vi "AlliGator Register Control Events.vi"(8 "Error In":errorcluster, 11 "AlliGator Control References":T2) -> (0 "Error Out":errorcluster, 3 "AlliGator Events Registration":T1)   [LabVIEW 2021, in "AlliGator GUI.lvlib"]
doc: "Registers user events for controls on the main AlliGator window."
uses:
  AlliGator GUI.lvlib
  AlliGator Registered Events Ctrl Refnums.ctl
  AlliGator Events Registration.ctl
  Settings/AlliGator Settings Event.ctl
  Settings/AlliGator Settings Window Messages.ctl
  Phasor Plot Color Map/AlliGator Phasor Color Map User Event List.ctl
  Graphs/XY Graph/XY Graph Refnum.ctl
  Settings/AlliGator Settings.lvlib
  Phasor Plot Color Map/AlliGator Phasor Plot Color Map.lvlib
  Phasor Plot/AlliGator Phasor Plot.lvlib
  Graphs/XY Graph/XY Graph Add-Ons.lvlib
panel:
  # "see the AlliGator License on the block diagram (Ctrl+E or Window:Show Block Diagram)"
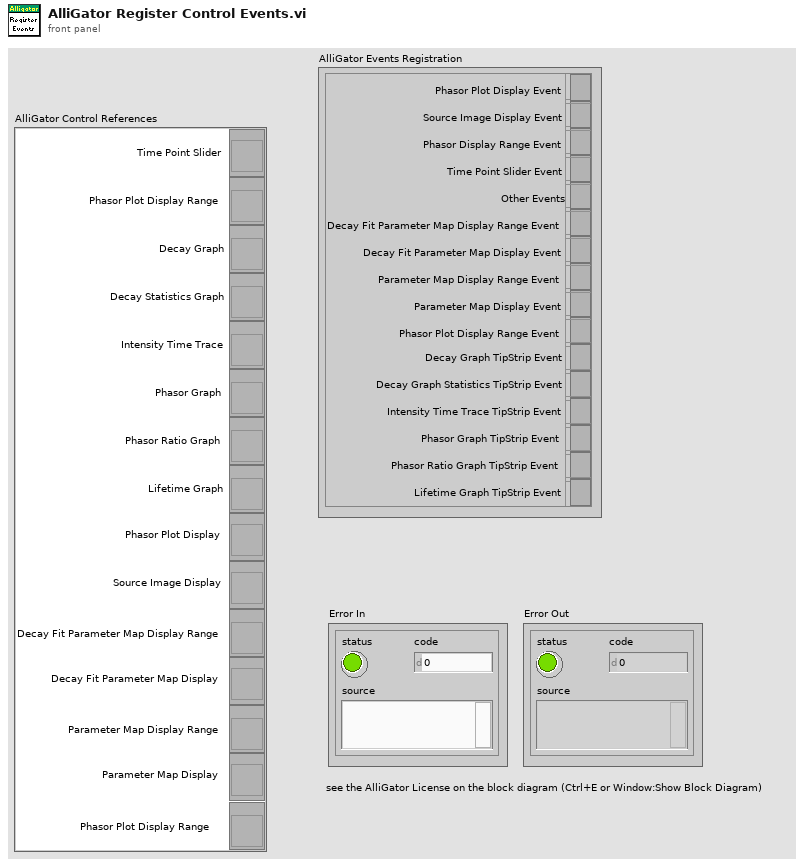
[diagram p1: front panel]
types:
  T1 = typedef "AlliGator GUI.lvlib/AlliGator Events Registration.ctl" = cluster{"Phasor Plot Display Event":refnum<event-registration>, "Source Image Display Event":refnum<event-registration>, "Phasor Display Range Event":refnum<event-registration>, "Time Point Slider Event":refnum<event-registration>, "Other Events":refnum<event-registration>, "Decay Fit Parameter Map Display Range Event":refnum<event-registration>, "Decay Fit Parameter Map Display Event":refnum<event-registration>, "Parameter Map Display Range Event":refnum<event-registration>, "Parameter Map Display Event":refnum<event-registration>, "Phasor Plot Display Range Event":refnum<event-registration>, "Decay Graph TipStrip Event":refnum<event-registration>, "Decay Graph Statistics TipStrip Event":refnum<event-registration>, "Intensity Time Trace TipStrip Event":refnum<event-registration>, "Phasor Graph TipStrip Event":refnum<event-registration>, "Phasor Ratio Graph TipStrip Event":refnum<event-registration>, "Lifetime Graph TipStrip Event":refnum<event-registration>}
  T2 = typedef "AlliGator GUI.lvlib/AlliGator Registered Events Ctrl Refnums.ctl" = cluster{"Time Point Slider":refnum<vi>, "Phasor Plot Display Range":refnum<vi>, "Decay Graph":refnum<vi>, "Decay Statistics Graph":refnum<vi>, "Intensity Time Trace":refnum<vi>, "Phasor Graph":refnum<vi>, "Phasor Ratio Graph":refnum<vi>, "Lifetime Graph":refnum<vi>, "Phasor Plot Display":refnum<vi>, "Source Image Display":refnum<vi>, "Decay Fit Parameter Map Display Range":refnum<vi>, "Decay Fit Parameter Map Display":refnum<vi>, "Parameter Map Display Range":refnum<vi>, "Parameter Map Display":refnum<vi>, "Phasor Plot Display Range":refnum<vi>}
  T3 = cluster{"Event Registration Refnum":refnum<event-registration>, "Event Registration Refnum":refnum<event-registration>, "Event Registration Refnum":refnum<event-registration>, "Event Registration Refnum":refnum<event-registration>, "Event Registration Refnum":refnum<event-registration>, "Event Registration Refnum":refnum<event-registration>, "Event Registration Refnum":refnum<event-registration>, "Event Registration Refnum":refnum<event-registration>, "Event Registration Refnum":refnum<event-registration>, "Event Registration Refnum":refnum<event-registration>, "Event Registration Refnum":refnum<event-registration>, "Event Registration Refnum":refnum<event-registration>, "Event Registration Refnum":refnum<event-registration>, "Event Registration Refnum":refnum<event-registration>, "Event Registration Refnum":refnum<event-registration>, "Event Registration Refnum":refnum<event-registration>}
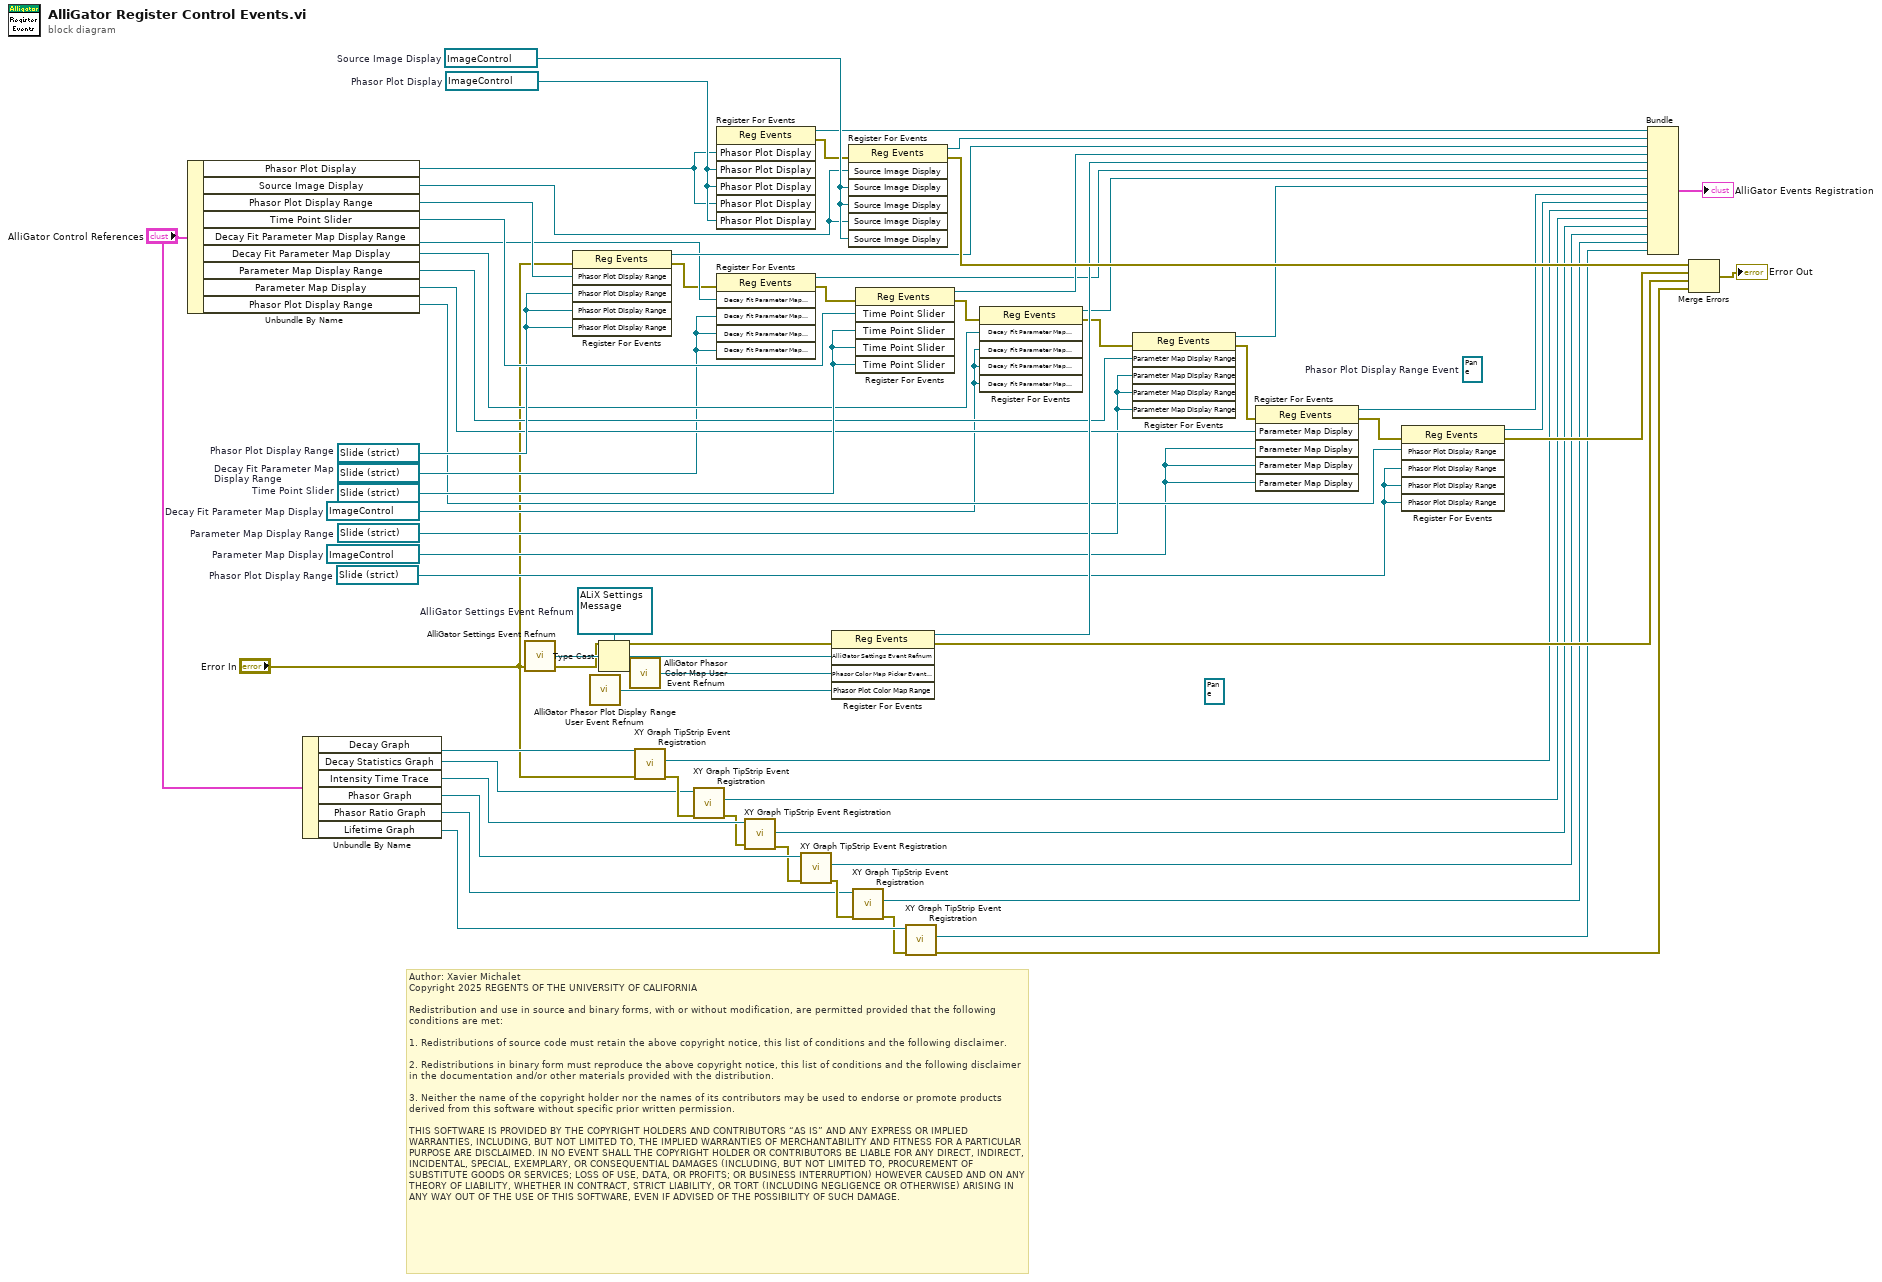
[diagram p0: block diagram]
diagram:
  (unwired) refnum<event-registration> refnum ("Decay Graph TipStrip Event")
  (unwired) refnum<event-registration> refnum  # Phasor Plot Display Range Event
  w25 = refnum<vi> refnum  # Phasor Plot Display Range
  w23 = refnum<vi> refnum  # Parameter Map Display
  w31 = refnum<vi> refnum  # Parameter Map Display Range
  w22 = refnum<vi> refnum  # Decay Fit Parameter Map Display
  w32 = refnum<vi> refnum  # Decay Fit Parameter Map Display Range
  w47 = refnum<vi> refnum  # Time Point Slider
  w48 = refnum<vi> refnum  # Phasor Plot Display Range
  w66 = refnum<user-event> refnum  # AlliGator Settings Event Refnum
  w62 = refnum<vi> refnum  # Source Image Display
  w63 = refnum<vi> refnum  # Phasor Plot Display
  # "Author: Xavier Michalet\nCopyright 2025 REGENTS OF THE UNIVERSITY OF CALIFORNIA\n\nRedistribution and use in source and binary forms, with or without modification, are permitted provided that the following conditions are met:\n\n1. Redistributions of source code must retain the above copyright notice, this list of conditions and the following disclaimer.\n\n2. Redistributions in binary form must reproduce the above copyright notice, this list of conditions and the following disclaimer in the documentation and/or other materials provided with the distribution.\n\n3. Neither the name of the copyright holder nor the names of its contributors may be used to endorse or promote products derived from this software without specific prior written permission.\n\nTHIS SOFTWARE IS PROVIDED BY THE COPYRIGHT HOLDERS AND CONTRIBUTORS “AS IS” AND ANY EXPRESS OR IMPLIED WARRANTIES, INCLUDING, BUT NOT LIMITED TO, THE IMPLIED WARRANTIES OF MERCHANTABILITY AND FITNESS FOR A PARTICULAR PURPOSE ARE DISCLAIMED. IN NO EVENT SHALL THE COPYRIGHT HOLDER OR CONTRIBUTORS BE LIABLE FOR ANY DIRECT, INDIRECT, INCIDENTAL, SPECIAL, EXEMPLARY, OR CONSEQUENTIAL DAMAGES (INCLUDING, BUT NOT LIMITED TO, PROCUREMENT OF SUBSTITUTE GOODS OR SERVICES; LOSS OF USE, DATA, OR PROFITS; OR BUSINESS INTERRUPTION) HOWEVER CAUSED AND ON ANY THEORY OF LIABILITY, WHETHER IN CONTRACT, STRICT LIABILITY, OR TORT (INCLUDING NEGLIGENCE OR OTHERWISE) ARISING IN ANY WAY OUT OF THE USE OF THIS SOFTWARE, EVEN IF ADVISED OF THE POSSIBILITY OF SUCH DAMAGE."
  n1 = Unbundle By Name("AlliGator Control References") -> ("Phasor Plot Display"=w40:refnum<vi>, "Source Image Display"=w41:refnum<vi>, "Phasor Plot Display Range"=w52:refnum<vi>, "Time Point Slider"=w50:refnum<vi>, "Decay Fit Parameter Map Display Range"=w45:refnum<vi>, "Decay Fit Parameter Map Display"=w38:refnum<vi>, "Parameter Map Display Range"=w34:refnum<vi>, "Parameter Map Display"=w35:refnum<vi>, "Phasor Plot Display Range"=w26:refnum<vi>)
  n2 = Unbundle By Name("AlliGator Control References") -> ("Decay Graph"=w20:refnum<vi>, "Decay Statistics Graph"=w15:refnum<vi>, "Intensity Time Trace"=w14:refnum<vi>, "Phasor Graph"=w13:refnum<vi>, "Phasor Ratio Graph"=w9:refnum<vi>, "Lifetime Graph"=w8:refnum<vi>)
  n3 = call "AlliGator Settings Event Refnum.vi"("Error In"="Error In") -> ("AlliGator Settings Event Refnum"=w65:refnum<user-event>, "Error Out"=w46:errorcluster)  [unwired: 7 in]
  n4 = register-events(error in="Error In", w52, w48, w48, w48) -> (reference out=w51:refnum<event-registration>, error out=w44:errorcluster)  [unwired: 1 in]
  n5 = call "AlliGator Phasor Plot Display Range User Event Refnum.vi"() -> ("Phasor Plot Color Map Range"=w57:refnum<user-event>)  [unwired: 9 in]
  n6 = Type Cast(type=w66, x=w65) -> (*(type *) &x=w59:refnum<user-event>)
  n7 = call "AlliGator Phasor Color Map User Event Refnum.vi"() -> ("Phasor Color Map Picker Event Refnum"=w58:refnum<user-event>)  [unwired: 9 in]
  n8 = call "XY Graph TipStrip Event Registration.vi"("error in (no error)"="Error In", "XY Graph Refnum"=w20) -> ("error out"=w16:errorcluster, "Event Registration Refnum"=w18:refnum<event-registration>)  [unwired: 7 in, 1 out]
  n9 = call "XY Graph TipStrip Event Registration.vi"("error in (no error)"=w16, "XY Graph Refnum"=w15) -> ("error out"=w12:errorcluster, "Event Registration Refnum"=w5:refnum<event-registration>)  [unwired: 7 in, 1 out]
  n10 = register-events(w40, w63, w63, w40, w63) -> (reference out=w61:refnum<event-registration>, error out=w54:errorcluster)  [unwired: 2 in]
  n11 = register-events(error in=w44, w45, w32, w32, w32) -> (reference out=w42:refnum<event-registration>, error out=w43:errorcluster)  [unwired: 1 in]
  n12 = call "XY Graph TipStrip Event Registration.vi"("error in (no error)"=w12, "XY Graph Refnum"=w14) -> ("error out"=w11:errorcluster, "Event Registration Refnum"=w4:refnum<event-registration>)  [unwired: 7 in, 1 out]
  n13 = call "XY Graph TipStrip Event Registration.vi"("error in (no error)"=w11, "XY Graph Refnum"=w13) -> ("error out"=w10:errorcluster, "Event Registration Refnum"=w3:refnum<event-registration>)  [unwired: 7 in, 1 out]
  n14 = register-events(error in=w46, w59, w58, w57) -> (reference out=w55:refnum<event-registration>, error out=w53:errorcluster)  [unwired: 1 in]
  n15 = register-events(error in=w54, w41, w62, w62, w41, w62) -> (reference out=w60:refnum<event-registration>, error out=w56:errorcluster)  [unwired: 1 in]
  n16 = call "XY Graph TipStrip Event Registration.vi"("error in (no error)"=w10, "XY Graph Refnum"=w9) -> ("error out"=w7:errorcluster, "Event Registration Refnum"=w2:refnum<event-registration>)  [unwired: 7 in, 1 out]
  n17 = register-events(error in=w43, w50, w47, w47, w47) -> (reference out=w49:refnum<event-registration>, error out=w39:errorcluster)  [unwired: 1 in]
  n18 = call "XY Graph TipStrip Event Registration.vi"("error in (no error)"=w7, "XY Graph Refnum"=w8) -> ("error out"=w6:errorcluster, "Event Registration Refnum"=w1:refnum<event-registration>)  [unwired: 7 in, 1 out]
  n19 = register-events(error in=w39, w38, w22, w22, w22) -> (reference out=w37:refnum<event-registration>, error out=w36:errorcluster)  [unwired: 1 in]
  n20 = register-events(error in=w36, w34, w31, w31, w31) -> (reference out=w30:refnum<event-registration>, error out=w33:errorcluster)  [unwired: 1 in]
  n21 = register-events(error in=w33, w35, w23, w23, w23) -> (reference out=w29:refnum<event-registration>, error out=w28:errorcluster)  [unwired: 1 in]
  n22 = register-events(error in=w28, w26, w25, w25, w25) -> (reference out=w24:refnum<event-registration>, error out=w27:errorcluster)  [unwired: 1 in]
  n23 = Bundle("Event Registration Refnum"=w61, "Event Registration Refnum"=w60, "Event Registration Refnum"=w51, "Event Registration Refnum"=w49, "Event Registration Refnum"=w55, "Event Registration Refnum"=w42, "Event Registration Refnum"=w37, "Event Registration Refnum"=w30, "Event Registration Refnum"=w29, "Event Registration Refnum"=w24, "Event Registration Refnum"=w18, "Event Registration Refnum"=w5, "Event Registration Refnum"=w4, "Event Registration Refnum"=w3, "Event Registration Refnum"=w2, "Event Registration Refnum"=w1) -> (→"AlliGator Events Registration":T3)  [unwired: 1 in]
  n24 = Merge Errors(w56, w27, w53, w6) -> (→"Error Out":errorcluster)
